vi "Get Location of next IFD from file.vi"(5 "Litt/BigEnd":bool, 6 "error in":errorcluster, 7 "Start of current IFD\n(ImFileDirectOffs)":u32, 9 "File":refnum<file>) -> (0 "error out":errorcluster, 1 "Location in byte stream of \nLong Word that points to this next IFD":u32, 2 "Location in byte stream of \nnext IFD if there is a next IFD,\n0 otherwise":u32, 3 "File out":refnum<file>, 4 "# of tags":u16)   [LabVIEW 2015, in "Tiff reader.lvlib"]
doc: "Obtains the location of the pointer that points to the next IFD location. It also returns the destination of the pointer, the location of the next IFD. This is done via accessing the file on disk."
uses:
  Tiff reader.lvlib
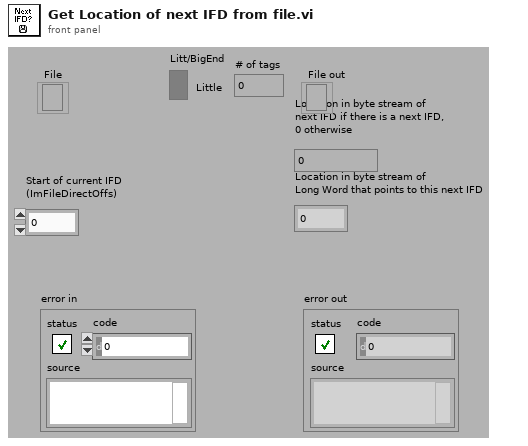
[diagram p1: front panel]
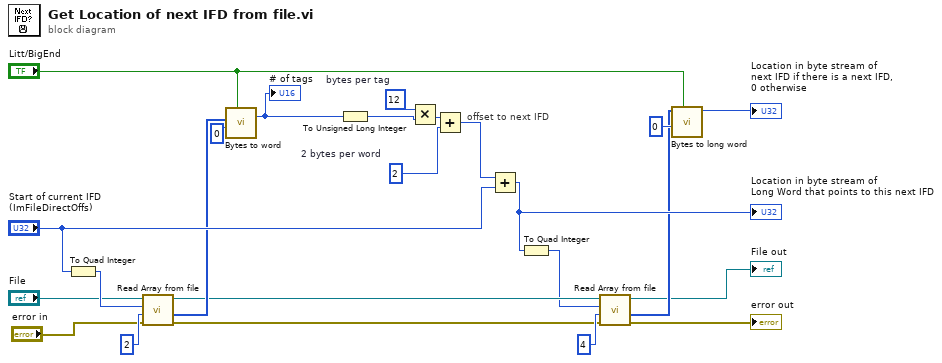
[diagram p0: block diagram]
diagram:
  w19 = u32 2  # 2 bytes per word
  w20 = u32 12  # bytes per tag
  # "offset to next IFD"
  n1 = To Quad Integer(1:"Start of current IFD\n(ImFileDirectOffs)") -> (0:w12:i64)
  n2 = call "Read Array from file.vi"("error in"="error in", "bytes to read"=2, "File location in"=w12, "File"="File") -> ("error out"=w4:errorcluster, "Array of U8s"=w10:u8[], "File out"=w6:refnum<file>)  [unwired: 1 out]
  n3 = call "Bytes to word.vi"("Litt/BigEnd"="Litt/BigEnd", "Index"=0, "Image Data in"=w10) -> ("Word"=w18:u16)  [unwired: 1 in, 5 out]
  "# of tags" <- w18
  n4 = To Unsigned Long Integer(number=w18) -> (unsigned 32bit integer=w17:u32)
  n5 = Multiply(x=w20, y=w17) -> (x*y=w21:u32)
  n6 = Add(x=w21, y=w19) -> (x+y=w22:u32)
  n7 = Add(x=w22, y="Start of current IFD\n(ImFileDirectOffs)") -> (x+y=w14:u32)
  "Location in byte stream of \nLong Word that points to this next IFD" <- w14
  n8 = To Quad Integer(1:w14) -> (0:w5:i64)
  n9 = call "Read Array from file.vi"("error in"=w4, "bytes to read"=4, "File location in"=w5, "File"=w6) -> ("error out"=→"error out":errorcluster, "Array of U8s"=w2:u8[], "File out"=→"File out":refnum<file>)  [unwired: 1 out]
  n10 = call "Bytes to long word.vi"("Litt/BigEnd"="Litt/BigEnd", "Index"=0, "Image Data in"=w2) -> ("U32"=→"Location in byte stream of \nnext IFD if there is a next IFD,\n0 otherwise":u32)  [unwired: 6 out]
